vi "Ease to a Stop.vi"() -> ()   [LabVIEW 2011, in "Sliding Menu Library.lvlib" / "Sliding Menu XControl.xctl"]
uses:
  Sliding Menu xControl/Sliding Menu XControl.xctl
panel:
  out "error out":errorcluster
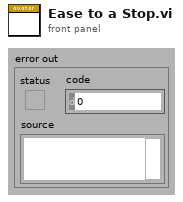
[diagram p1: front panel]
types:
  T1 = typedef "Sliding Menu Library.lvlib/Sliding Menu XControl.xctl/Sliding Menu State.ctl" = cluster{"Numeric":dbl, "Array of Button References":refnum<vi>[], "Space Between Menu Buttons":i32, "Number of Menu Buttons":i32, "Array of Button Names":string[], "Most Recent Vertical Position":i32, "This VI":refnum<vi>, "Current Action":T2, "Most Recent Distance Traveled":i32, "Method":T3, "Data In":T4}
  T2 = typedef "Sliding Menu Library.lvlib/Current User Action.ctl" = enum16{"Not Moving", "Mouse Down", "Mouse Up No Dragging", "Bounce Up Needed", "Bounce Down Needed", "Dragging", "Easing"}
  T3 = typedef "Sliding Menu Methods.ctl" = enum16{"Resize", "Move Up", "Move Down", "Move to 0"}
  T4 = typedef "Sliding Menu Library.lvlib/Sliding Menu XControl.xctl/Sliding Menu Data.ctl" = i32
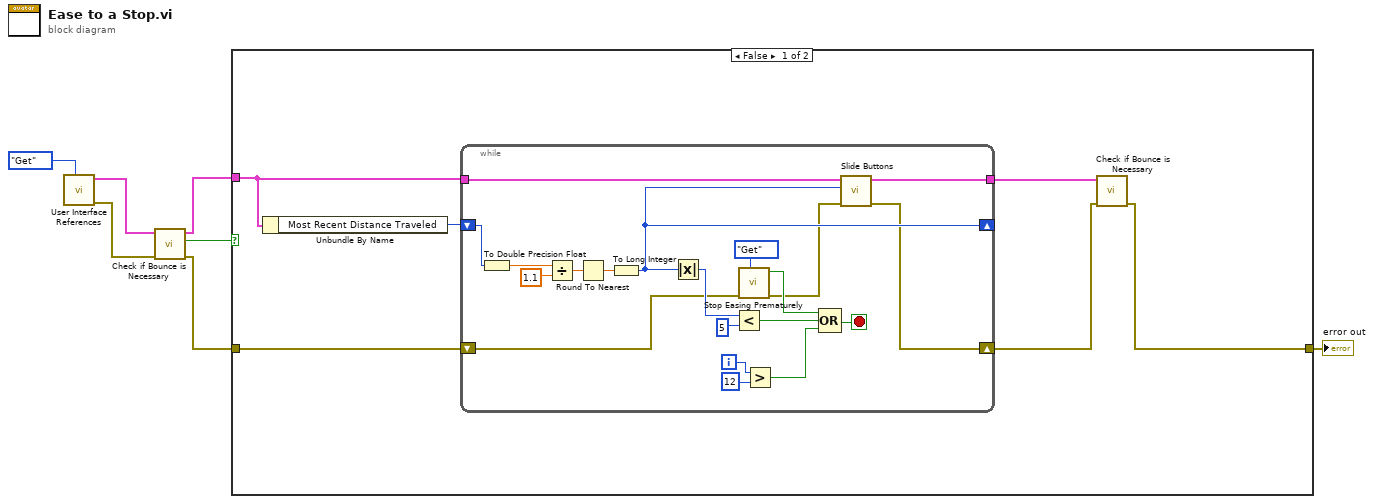
[diagram p0: block diagram]
diagram:
  n1 = call "User Interface References.vi"("Set or Get Value"=enum16{"Set", "Get"}."Get") -> ("error out"=w5:errorcluster, "Display State Out"=w6:T1)  [unwired: 9 in]
  n2 = call "Check if Bounce is Necessary.vi"("error in"=w5, "Display State In"=w6) -> ("error out"=w2:errorcluster, "Was Bounce Done?"=w4:bool, "Display State Out 2"=w3:T1)  [unwired: 7 in]
  n3 = case shown="False" w4 {
    tunnel: w3 -> [w13 _]
    tunnel: w2 -> [w11 w34]
    tunnel: [w8 w34] -> w1
    frame False {
      n4 = Unbundle By Name(w13) -> ("Most Recent Distance Traveled"=w12:i32)
      n5 = while {
        tunnel: w13 -> [w33]
        shift-right: [w20] -> w9
        shift-left: w11 -> [w15]
        shift-right: [w25] -> _
        shift-left: w12 -> [w26]
        tunnel: [w14] -> w10
        i -> [w23]
        stop <- w21 stop-if-true
        n6 = To Double Precision Float(number=w26) -> (double precision float=w32:dbl)
        n7 = Divide(x=w32, y=1.1) -> (x/y=w27:dbl)
        n8 = Round To Nearest(number=w27) -> (nearest integer value=w28:dbl)
        n9 = To Long Integer(number=w28) -> (32bit integer=w25:i32)
        n10 = Absolute Value(x=w25) -> (abs(x)=w29:i32)
        n11 = Less?(x=w29, y=5) -> (x < y?=w22:bool)
        n12 = call "Stop Easing Prematurely.vi"("Set or Get Value"=enum16{"Set", "Get"}."Get", "error in"=w15) -> ("error out"=w16:errorcluster, "Stop?"=w18:bool)  [unwired: 8 in]
        n13 = Greater?(x=w23, y=12) -> (0:w17:bool)
        n14 = Compound Arithmetic op=OR(w18, w22, w17) -> (w21:bool)
        n15 = call "Slide Buttons.vi"("error in (no error)"=w16, "Distance"=w25, "Display State In"=w33) -> ("error out"=w20:errorcluster, "Display State Out"=w14:T1)  [unwired: 7 in]
      }
      n16 = call "Check if Bounce is Necessary.vi"("error in"=w9, "Display State In"=w10) -> ("error out"=w8:errorcluster)  [unwired: 7 in, 2 out]
    }
    frame True {
    }
  }
  "error out" <- w1
